vi "Delete Last Element.vi"(8 "error in (no error)":errorcluster, 11 "Variant in":variant) -> (0 "error out":errorcluster, 3 "Variant out":variant, 9 "element":variant, 10 "Name":string)   [LabVIEW 2017, in "Advanced Variant Tools.lvlib" / "Data Manipulation.lvlib"]
uses:
  Data Manipulation.lvlib
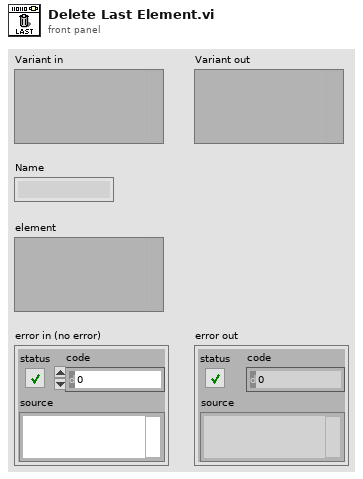
[diagram p1: front panel]
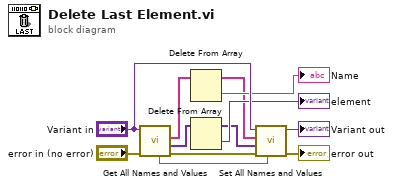
[diagram p0: block diagram]
diagram:
  n1 = call "Get All Names and Values.vi"("error in"="error in (no error)", "Cluster In"="Variant in") -> ("error out"=w10:errorcluster, "Values"=w11:variant[], "Item Names"=w6:string[], "Name"=w1:string)  [unwired: 5 in, 1 out]
  n2 = Delete From Array(array=w6) -> (deleted portion=→"Name":string, array with subset deleted=w3:string[])  [unwired: 2 in]
  n3 = Delete From Array(array=w11) -> (deleted portion=→"element":variant, array with subset deleted=w2:variant[])  [unwired: 2 in]
  n4 = call "Set All Names and Values.vi"("Name"=w1, "error in"=w10, "values"=w2, "Item Names"=w3, "Cluster In"="Variant in") -> ("error out"=→"error out":errorcluster, "Cluster Out"=→"Variant out":variant)  [unwired: 5 in]
